vi "ClimbGlobals.vi"() -> ()   [LabVIEW 2020]
panel:
  in  "ClimbButton":i32
  in  "ClimbState":i32
  in  "Arm2Extended":bool
  in  "Arm1Extended":bool
  in  "ArmForward":bool
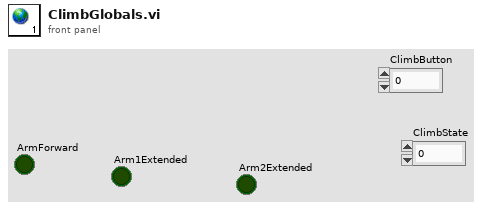
[diagram p1: front panel]
diagram:
